vi "C DLL.vi"(0 "Input1":dbl, 5 "Input2":dbl, 7 "Arithmetic Operation":string(combo)) -> (4 "Output":dbl)   [LabVIEW 2020, in "LV Connectivity.lvlib"]
doc: "This VI is used as a C DLL to perform basic arithmetic operation whihc can be called as librray by another module to perform the required operation."
uses:
  LV Connectivity.lvlib
panel:
  # "C DLL"
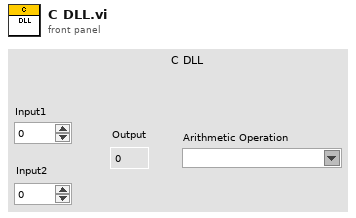
[diagram p1: front panel]
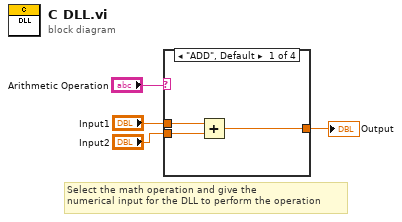
[diagram p0: block diagram]
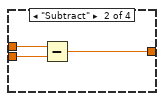
[diagram p2: hidden frame]
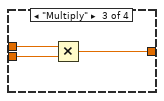
[diagram p3: hidden frame]
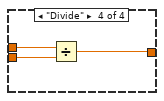
[diagram p4: hidden frame]
diagram:
  # "Select the math operation and give the \nnumerical input for the DLL to perform the operation"
  n1 = case shown="\"ADD\", Default" "Arithmetic Operation" {
    tunnel: "Input1" -> [w7 w10 w13 w16]
    tunnel: "Input2" -> [w6 w9 w12 w15]
    tunnel: [w5 w8 w11 w14] -> w2
    frame "ADD", Default {
      n2 = Add(x=w7, y=w6) -> (x+y=w5:dbl)
    }
    frame "Subtract" {
      n3 = Subtract(x=w10, y=w9) -> (x-y=w8:dbl)
    }
    frame "Multiply" {
      n4 = Multiply(x=w13, y=w12) -> (x*y=w11:dbl)
    }
    frame "Divide" {
      n5 = Divide(x=w16, y=w15) -> (x/y=w14:dbl)
    }
  }
  "Output" <- w2
